vi "Synchronize.vi"(7 "Retries (3)":i32=3, 8 "Error In":errorcluster, 11 "LINX Device Config":T1) -> (0 "Error Out":errorcluster, 3 "LINX Device Config":T1)   [LabVIEW 2016, in "LMH-LINX.lvlib" / "Device.lvlib"]
doc: "Synchronize the LINX device with LabVIEW."
uses:
  <vilib>/MakerHub/LINX/Private/Device/Device.lvlib
  <vilib>/MakerHub/LINX/Private/Device/Type Defs/LINX Device Config.ctl
  <vilib>/MakerHub/LINX/Private/Type Defs/Interface.ctl
  <vilib>/MakerHub/LINX/Private/Device/Type Defs/TCP Config.ctl
  <vilib>/MakerHub/LINX/Private/Device/Type Defs/Channels.ctl
  <vilib>/MakerHub/LINX/Private/Type Defs/Error Type.ctl
  <vilib>/MakerHub/LINX/LMH-LINX.lvlib
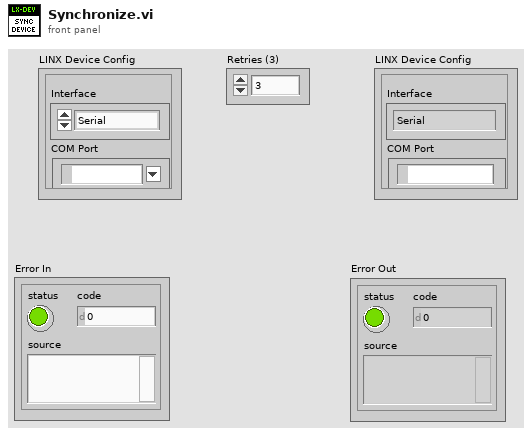
[diagram p1: front panel]
types:
  T1 = typedef "LMH-LINX.lvlib/Device.lvlib/LINX Device Config.ctl" = cluster{"Interface":T2, "COM Port":refnum<visa-resource-name>, "TCP Configuration":T3, "Device Family":u8, "Device ID":u8, "Device Name":string, "TCP Ref":refnum<k5>, "Channels":T4}
  T2 = typedef "LMH-LINX.lvlib/Interface.ctl" = enum16{"Serial", "TCP"}
  T3 = typedef "LMH-LINX.lvlib/Device.lvlib/TCP Config.ctl" = cluster{"IP Address":string, "Port":u16}
  T4 = typedef "LMH-LINX.lvlib/Channels.ctl" = cluster{"DI":u8[], "DO":u8[], "AI":u8[], "AO":u8[], "PWM":u8[], "QE":u8[], "UART":u8[], "I2C 2":u8[], "SPI":u8[], "CAN":u8[], "Servo":u8[], "AI Ref (V)":dbl, "AI Resolution (Bits)":u8, "AO Ref (V)":dbl, "AO Resolution (Bits)":u8}
  T5 = typedef "LMH-LINX.lvlib/Error Type.ctl" = enum16{"Unknown", "Timeout", "Corrupt Return Packet", "Unable To Connect", "Command Not Supported", "Channel DNE", "Invalid COM Config", "Firmware Version Mismatch", "myRIO Support", "CMD Specific Error", "Local IO Not Supported"}
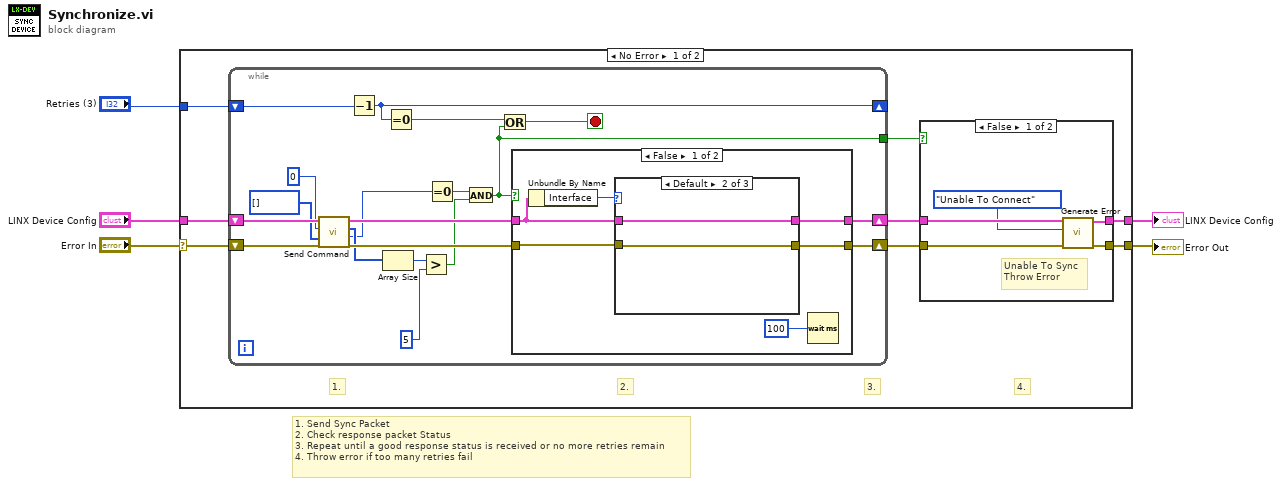
[diagram p0: block diagram]
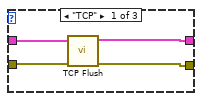
[diagram p3: hidden frame]
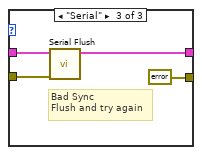
[diagram p4: hidden frame]
diagram:
  # "1. Send Sync Packet\n2. Check response packet Status\n3. Repeat until a good response status is received or no more retries remain\n4. Throw error if too many retries fail"
  n1 = case shown="No Error" "Error In" {
    selector: "Error In" -> [w6 w59]
    tunnel: "Retries (3)" -> [w13 _]
    tunnel: "LINX Device Config" -> [w12 w58]
    tunnel: [w8 w58] -> w3
    tunnel: [w7 w59] -> w2
    frame No Error {
      # "4."
      # "3."
      # "2."
      # "1."
      n2 = while {
        shift-right: [w34] -> _
        shift-left: w13 -> [w35]
        shift-right: [w30] -> w10
        shift-left: w6 -> [w38]
        tunnel: [w22] -> w9
        shift-right: [w32] -> w11
        shift-left: w12 -> [w39]
        stop <- w28 stop-if-true
        n3 = call <vilib>:"Send Command.vi"("Error In"=w38, "ARGS"=u8[] [], "CMD"=u16 0, "LINX Device Config"=w39) -> ("Error Out"=w29:errorcluster, "Status"=w21:u8, "Response"=w27:u8[], "LINX Device Config"=w31:T1)  [unwired: 4 in]
        n4 = Decrement(x=w35) -> (x-1=w34:i32)
        n5 = Array Size(array=w27) -> (size(s)=w26:i32)
        n6 = Equal To 0?(x=w34) -> (x = 0?=w33:bool)
        n7 = Greater?(x=w26, y=5) -> (0:w24:bool)
        n8 = Equal To 0?(x=w21) -> (x = 0?=w23:bool)
        n9 = And(x=w23, y=w24) -> (x .and. y?=w22:bool)
        n10 = Or(x=w33, y=w22) -> (x .or. y?=w28:bool)
        n11 = case shown="False" w22 {
          tunnel: [w43 w57] -> w32
          tunnel: w31 -> [w42 w57]
          tunnel: [w40 w56] -> w30
          tunnel: w29 -> [w45 w56]
          frame False {
            n12 = Unbundle By Name(w42) -> ("Interface"=w41:T2)
            n13 = case shown="Default" w41 {
              tunnel: w42 -> [w49 w51 w55]
              tunnel: w45 -> [w46 w50 w54]
              tunnel: [w48 w51 w53] -> w43
              tunnel: [w47 w50 errorcluster {"status"=FALSE, "code"=0, "source"=""} ("Error Out")] -> w40
              frame "TCP" {
                n14 = call <vilib>:"TCP Flush.vi"("Error In"=w46, "LINX Device Config"=w49) -> ("Error Out"=w47:errorcluster, "LINX Device Config"=w48:T1)  [unwired: 7 in, 1 out]
              }
              frame Default {
              }
              frame "Serial" {
                # "Bad Sync\nFlush and try again"
                n15 = call <vilib>:"Serial Flush.vi"("Error In"=w54, "LINX Device Config"=w55) -> ("LINX Device Config"=w53:T1)  [unwired: 8 in, 1 out]
              }
            }
            n16 = Wait (ms)(milliseconds to wait=u32 100) -> ()  [unwired: 1 out]
          }
          frame True {
            # "Sync OK"
          }
        }
      }
      n17 = case shown="False" w9 {
        tunnel: [w18 w20] -> w8
        tunnel: w11 -> [w16 w20]
        tunnel: [w17 w19] -> w7
        tunnel: w10 -> [w14 w19]
        frame False {
          # "Unable To Sync\nThrow Error"
          n18 = call <vilib>:"Generate Error.vi"("Error In"=w14, "Error Type"=Error_Type."Unable To Connect", "LINX Device Config"=w16) -> ("Error Out"=w17:errorcluster, "Dup LINX Device Config"=w18:T1)  [unwired: 7 in]
        }
        frame True {
          # "Sync OK"
        }
      }
    }
    frame Error {
    }
  }
  "Error Out" <- w2
  "LINX Device Config" <- w3
